vi "ScannerInterfaceGetFGV.vi"(8 "error in":errorcluster, 9 "pie70 interface Set":string(combo)="7", 10 "FGV_Control":enum16{"Set", "Get"}(ring), 11 "pi517 Interface Set":string(combo)="5") -> (0 "error out":errorcluster, 2 "pi517 Interface Get":string, 3 "pie70 interface Get":string)   [LabVIEW 2010]
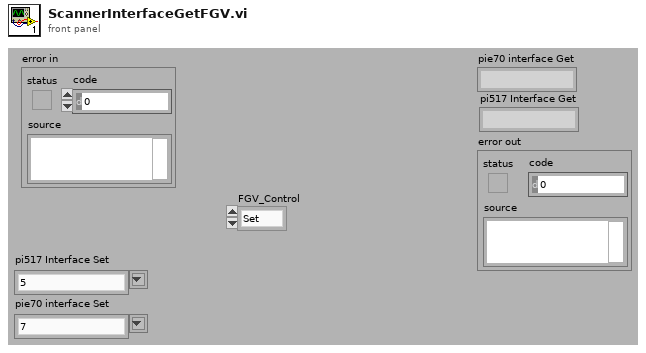
[diagram p1: front panel]
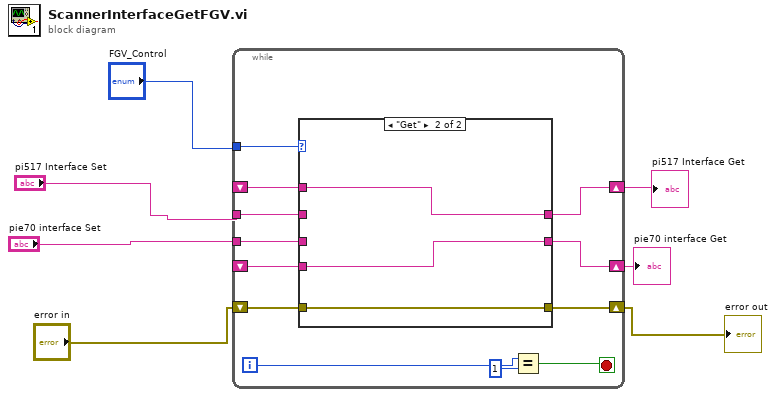
[diagram p0: block diagram]
diagram:
  n1 = while {
    tunnel: "FGV_Control" -> [w19]
    tunnel: "pi517 Interface Set" -> [w18]
    shift-right: [w17] -> w7
    shift-left: _ -> [w16]
    tunnel: "pie70 interface Set" -> [w12]
    shift-right: [w11] -> w4
    shift-left: _ -> [w10]
    shift-right: [w9] -> w2
    shift-left: "error in" -> [w8]
    i -> [w14]
    stop <- w15 stop-if-true
    n2 = case shown="\"Get\"" w19 {
      tunnel: w18 -> [w22 _]
      tunnel: [w22 w25] -> w17
      tunnel: w16 -> [_ w25]
      tunnel: w12 -> [w21 _]
      tunnel: [w21 w24] -> w11
      tunnel: w10 -> [_ w24]
      tunnel: w8 -> [w20 w23]
      tunnel: [w20 w23] -> w9
      frame "Set", Default {
      }
      frame "Get" {
      }
    }
    n3 = Equal?(x=w14, y=1) -> (x = y?=w15:bool)
  }
  "pie70 interface Get" <- w4
  "pi517 Interface Get" <- w7
  "error out" <- w2
